vi "Measurement UI.vi"() -> ()   [LabVIEW 2021, in "Stepped Frequency Sweep_Class D Amplifier.lvlib"]
uses:
  Stepped Frequency Sweep_Class D Amplifier.lvlib
panel:
  in  "Graphs":T1(tab)
  out "Time domain graph":waveform(dbl)(graph)
  out "Sweep graph":T2(graph)
  out "Frequency domain graph":T3(graph)
  out "Output power (W)":dbl[](array[numeric])
  out "SFDR (dB)":dbl[](array[numeric])
  out "Gain error (dB)":dbl[](array[numeric])
  out "Dynamic range (dB)":dbl[](array[numeric])
  out "THD (dB)":dbl[](array[numeric])
  out "THD+N (dB)":dbl[](array[numeric])
  out "SNR (dB)":dbl[](array[numeric])
  out "Calculated amplitude (dB)":dbl[](array[numeric])
  out "Calculated frequency (Hz)":dbl[](array[numeric])
  in  "Configuration tab":enum32{"Protocol", "Measurement"}(tab)
  in  "master clock channel list":string caption="Master Clock Channel"
  in  "digital channel list":string caption="Digital Audio Channel"
  in  "logic level":enum32{"3.3 V", "1.8 V", "1.2 V"}(ring) caption="Logic level"
  in  "master clock rate":dbl=12288000.0 caption="Master clock rate" format="%#_6pHz"
  out "Bit clock rate":dbl=3072000.0 format="%#_6pHz"
  in  "number of channels":u8=2 caption="Number of channels"
  in  "TDM":bool
  in  "RJ":bool
  in  "LJ":bool
  in  "I2S":bool
  in  "bit clock edge sync":enum32{"Rising", "Falling"}(ring)=enum."Falling" caption="Bit clock edge sync"
  in  "frame clock rate":dbl=48000.0 caption="Frame clock rate" format="%#_6pHz"
  in  "data justification":enum32{"Left Justified", "Right Justified"}(ring) caption="Data justification"
  in  "endianness":enum32{"MSB First", "LSB First"}(ring) caption="Endianness"
  in  "bit depth":u8=24 caption="Bit depth"
  in  "channel length":u16=32 caption="Channel length"
  in  "frame sync edge for channel 0":enum32{"Rising", "Falling"}(ring)=enum."Falling" caption="Frame sync edge for Channel 0"
  in  "min settling cycles":u32 caption="Minimum settling cycles"
  in  "min settling time (s)":dbl=0.1 caption="Minimum settling time" format="%#_6ps"
  in  "sweep profile":enum16{"Linear", "Logarithmic"}(ring)=enum."Logarithmic" caption="Profile"
  in  "number of steps":u32=20000 caption="Number of steps"
  in  "sweep start frequency (Hz)":dbl=20.0 caption="Sweep start" format="%#_6pHz"
  in  "sweep stop frequency (Hz)":dbl=20000.0 caption="Sweep stop" format="%#_6pHz"
  in  "output power (W)":dbl=1.0 caption="Output power" format="%#_6p W"
  in  "output mode":enum16{"Level", "Power"}(ring) caption="Output mode"
  in  "min measurement cycles":u32 caption="Minimum measurement cycles"
  in  "Acquisition channel":tag
  in  "acq sampling rate":dbl=51200.0 caption="Sample rate" format="%#.6pHz"
  in  "min measurement time (s)":dbl=0.1 caption="Minimum measurement time" format="%#_6ps"
  in  "lowpass filter":T4(ring) caption="Lowpass filter"
  in  "highpass filter":enum32{"DC", "AC"}(ring) caption="Highpass filter"
  in  "band start":dbl=20.0 caption="Band start" format="%#_6pHz"
  in  "band stop":dbl=20000.0 caption="Band stop" format="%#_6pHz"
  in  "weighting filter":T5(ring)=enum."A-weighting" caption="Weighting filter"
  in  "load impedance":dbl=4.0 caption="Load impedance" format="%#_6p Ohms"
  in  "output range (pk-pk)":dbl=15.0 caption="Output range" format="%.3p Vpk-pk"
  in  "output level (dB)":dbl=-1.0 caption="Output level" format="%#_6p dBFS"
  in  "channel 0 offset":u32=1
  out "fft - data":dbl[](array[numeric])
  out "fft - df":dbl
  out "fft - f0":dbl
  out "wfm - data":dbl[](array[numeric])
  out "wfm - dt":dbl
  out "wfm - t0":dbl
  out "Channel name":string
  in  "acq channel":string="PXI1Slot4/ai0"
  in  "signal phase":dbl caption="phase"
  # "hidden controls - used to sync with MeasLink"
  # "hidden indicators"
  # "Protocols"
  # "Audio Protocol"
  # "Clock Settings"
  # "Signal Level"
  # "Harware Resource"
  # "Sweep"
  # "Filters"
  # "Output"
  # "Acquisition"
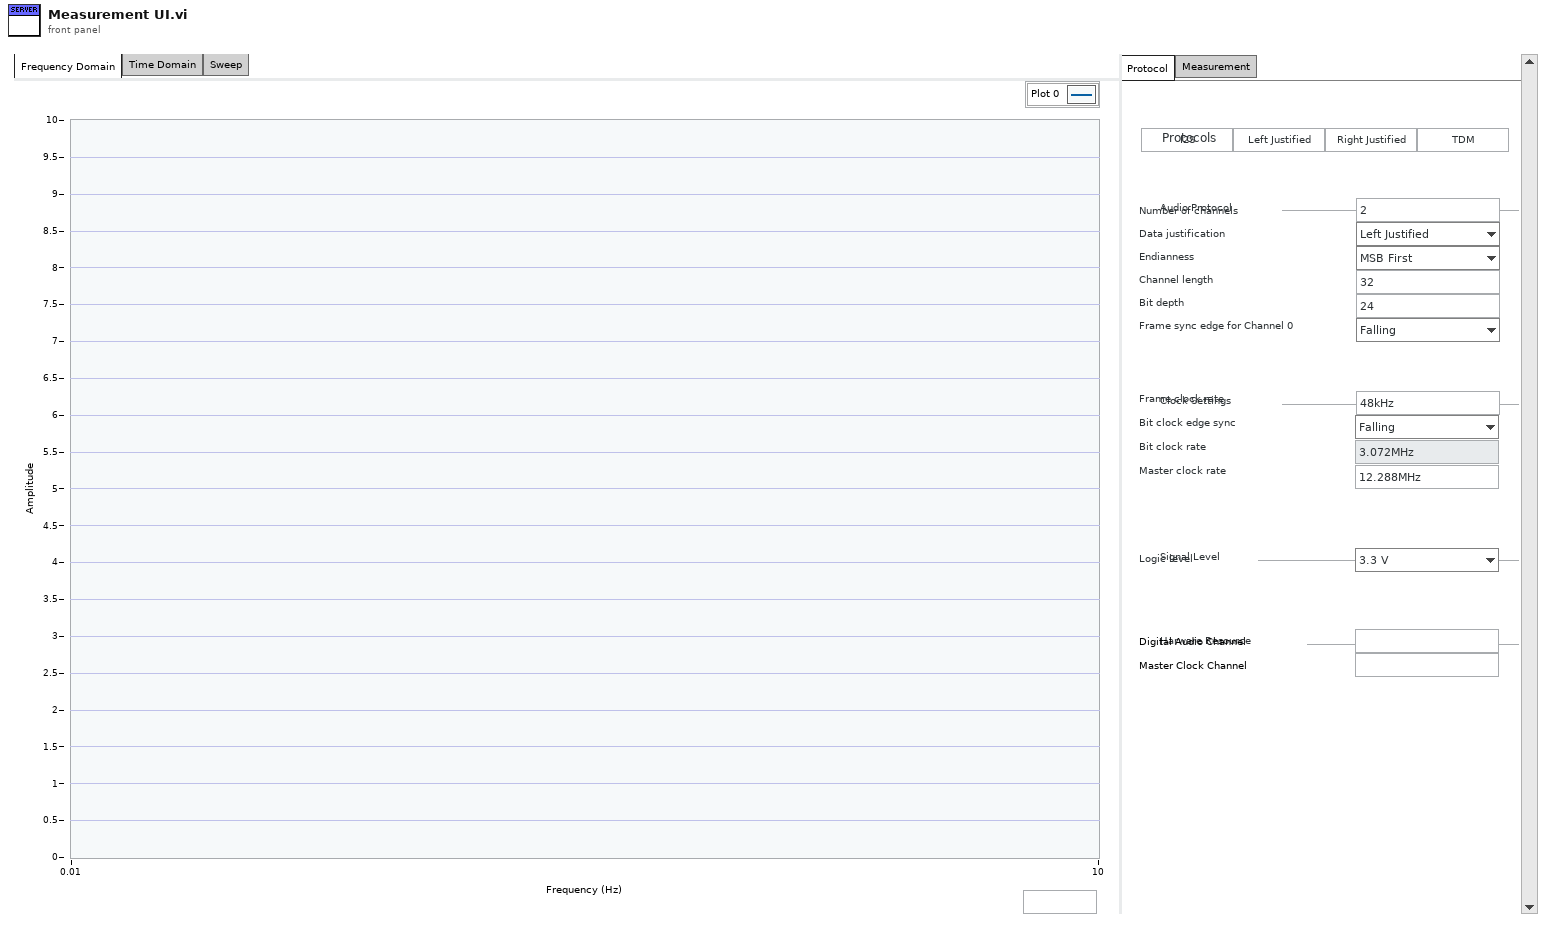
[diagram p1: front panel]
types:
  T1 = enum32{"Frequency Domain", "Time Domain", "Sweep"}
  T2 = cluster{"Calculated frequency (Hz)":dbl[], "THD+N (dB)":dbl[]}
  T3 = cluster{"fft - f0":dbl, "fft - df":dbl, "fft - data":dbl[]}
  T4 = enum32{"No filter", "AES17 20kHz", "AES17 40kHz"}
  T5 = enum32{"Linear", "A-weighting", "B-weighting", "C-weighting"}
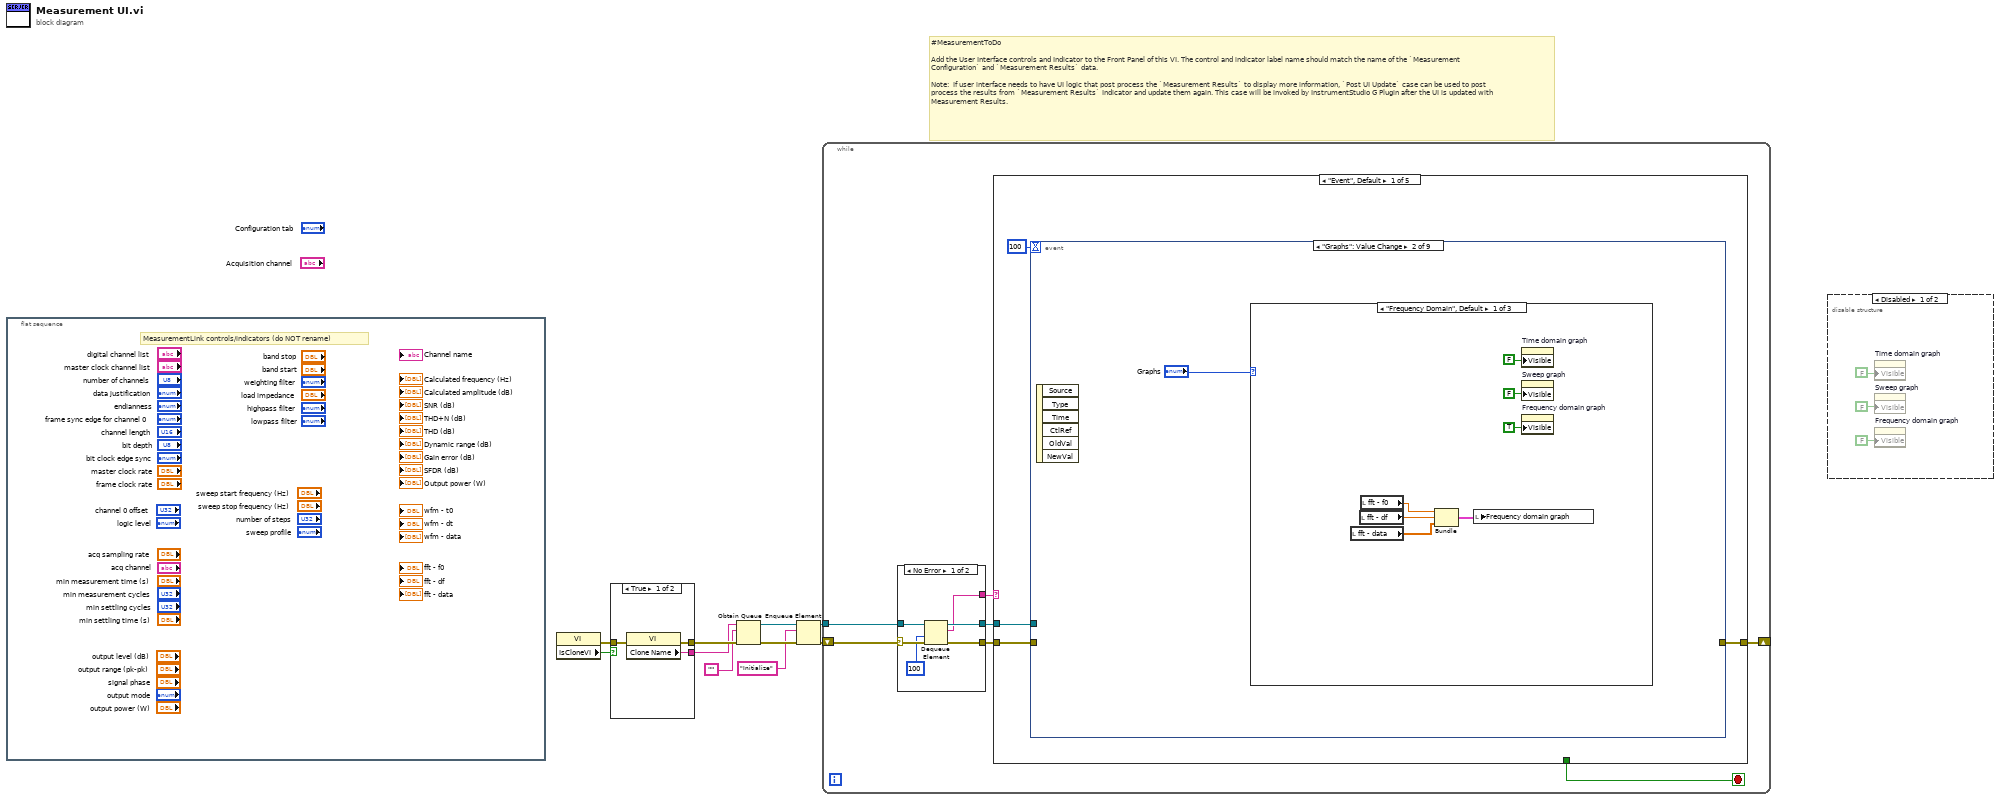
[diagram p0: block diagram]
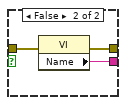
[diagram p3: hidden frame]
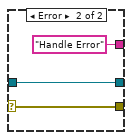
[diagram p4: hidden frame]
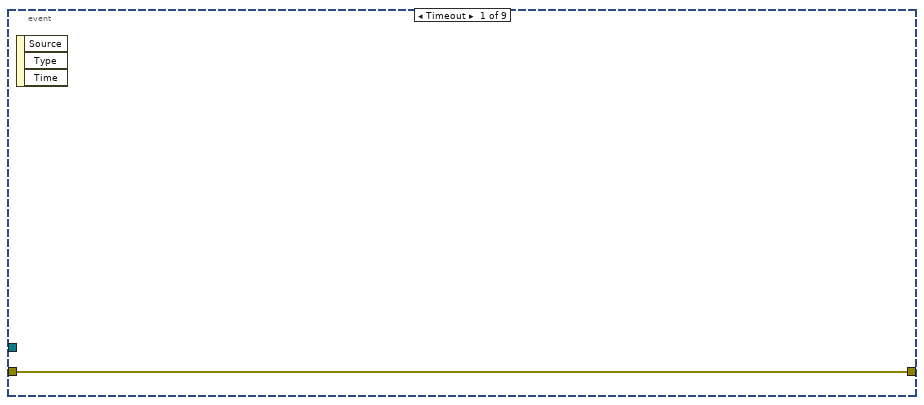
[diagram p5: hidden frame]
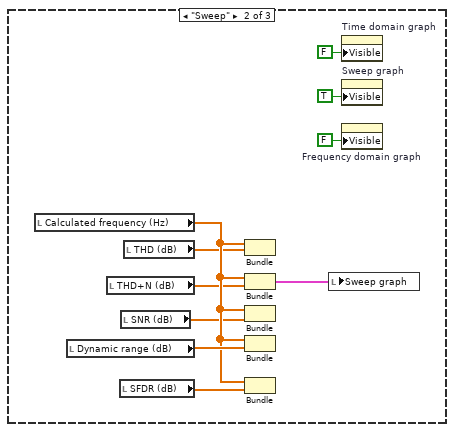
[diagram p6: hidden frame]
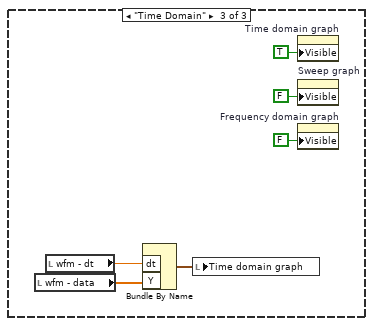
[diagram p7: hidden frame]
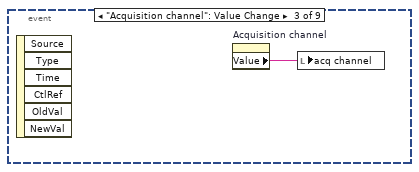
[diagram p8: hidden frame]
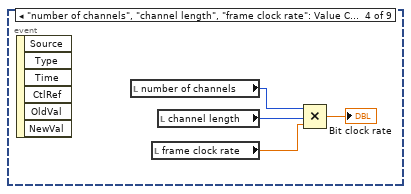
[diagram p9: hidden frame]
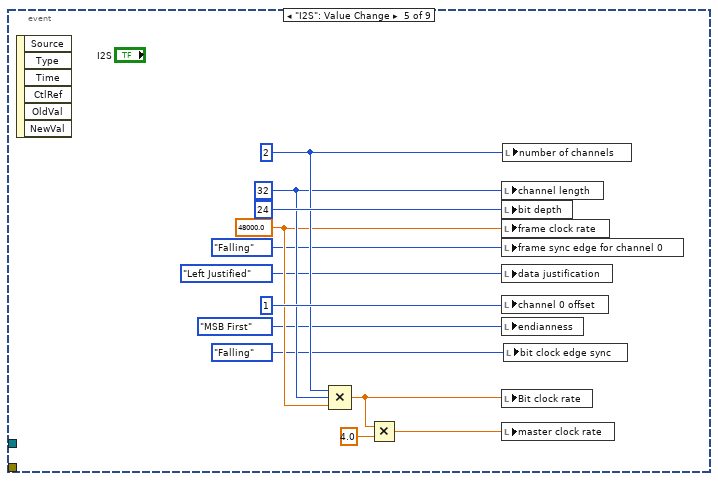
[diagram p10: hidden frame]
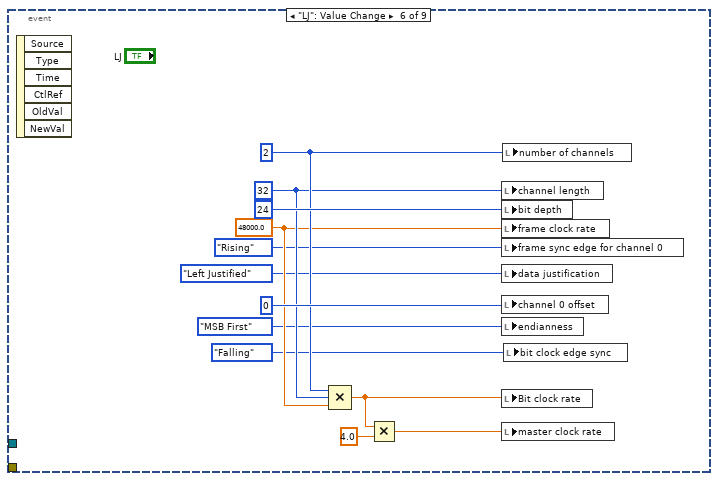
[diagram p11: hidden frame]
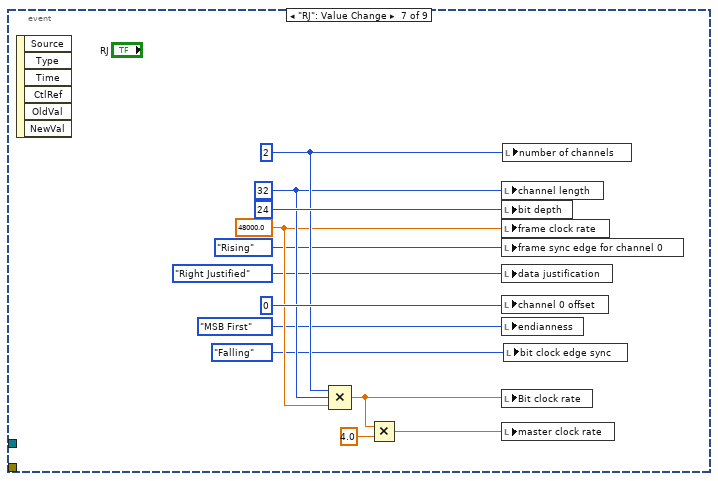
[diagram p12: hidden frame]
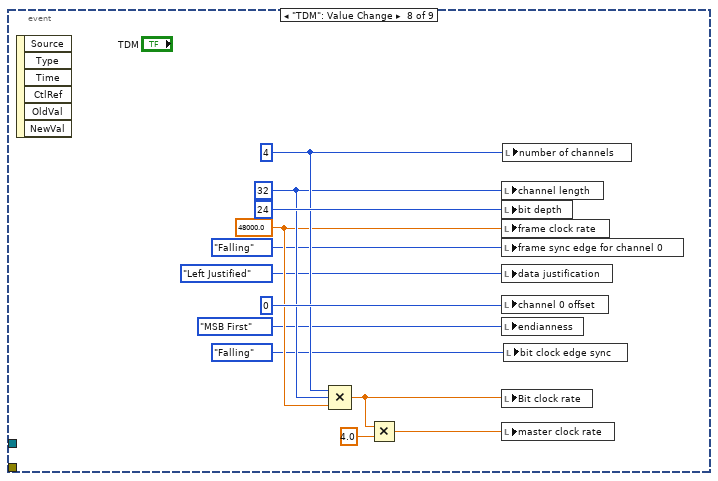
[diagram p13: hidden frame]
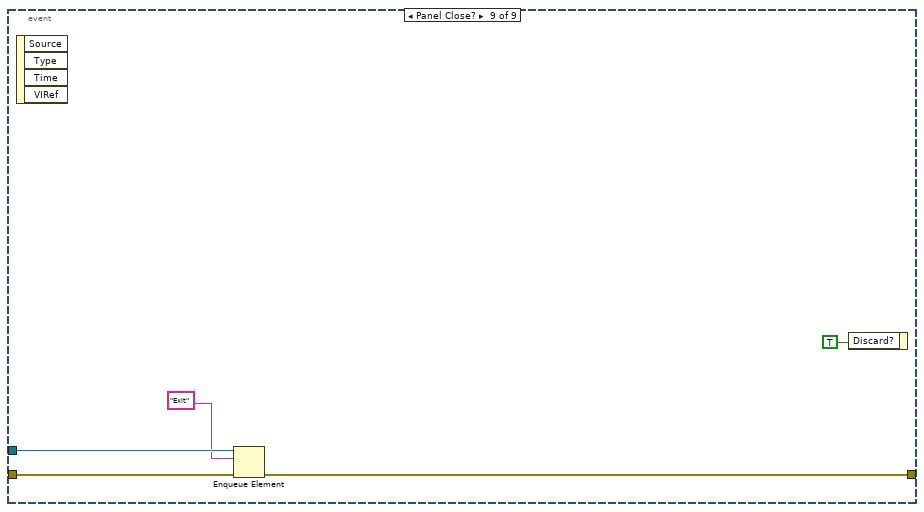
[diagram p14: hidden frame]
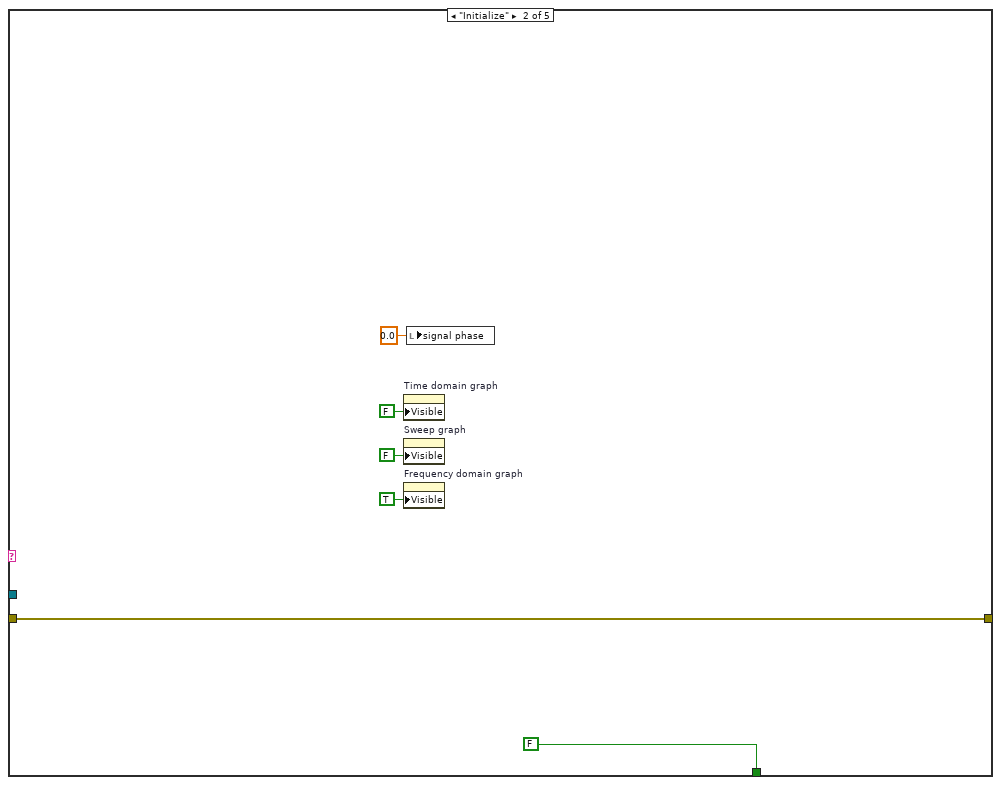
[diagram p15: hidden frame]
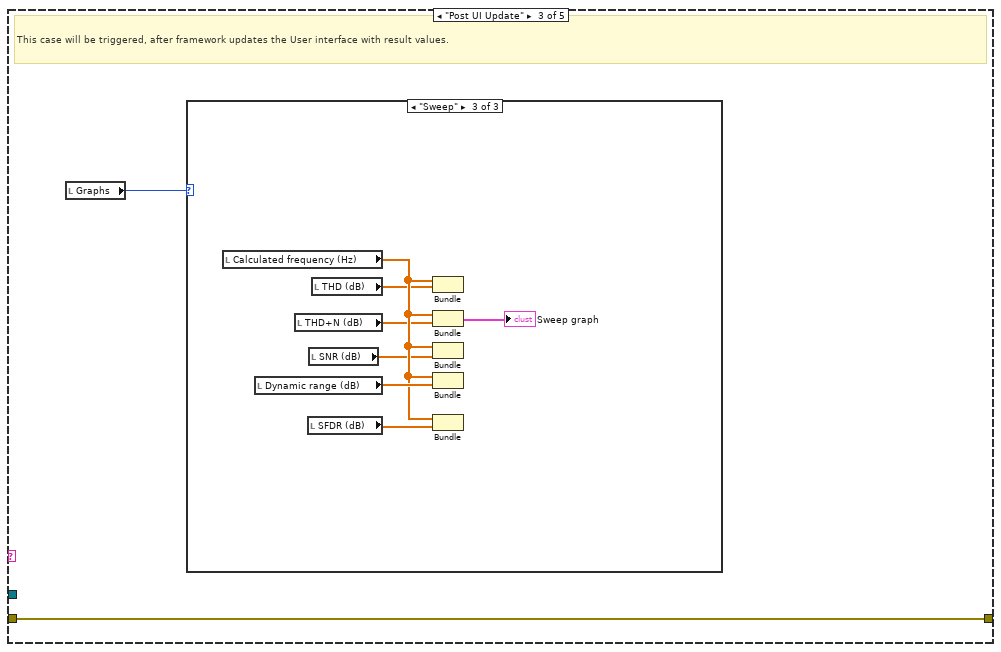
[diagram p16: hidden frame]
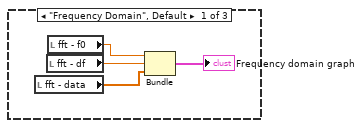
[diagram p17: hidden frame]
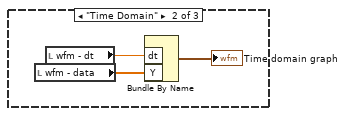
[diagram p18: hidden frame]
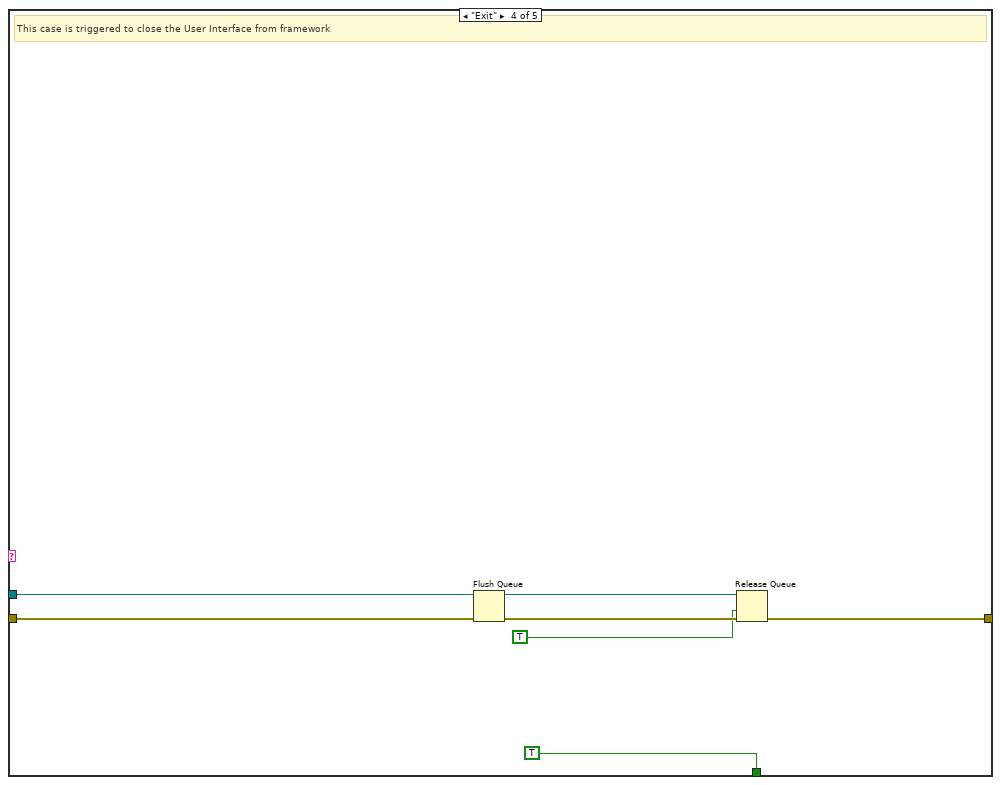
[diagram p19: hidden frame]
diagram:
  # "#MeasurementToDo  \n\nAdd the User Interface controls and Indicator to the Front Panel of this VI. The control and indicator label name should match the name of the `Measurement Configuration` and `Measurement Results` data.\n\nNote:  If user interface needs to have UI logic that post process the `Measurement Results` to display more information, `Post UI Update` case can be used to post process the results from `Measurement Results` Indicator and update them again. This case will be invoked by InstrumentStudio G Plugin after the UI is updated with Measurement Results."
  n1 = flat-sequence {
    frame #0 {
      # "MeasurementLink controls/indicators (do NOT rename)"
    }
  }
  n2 = property class="VI"() -> (error out=w1:errorcluster, "IsCloneVI"=w2:bool)  [unwired: 2 in, 1 out]
  n3 = case shown="True" w2 {
    tunnel: [w13 w16] -> w10
    tunnel: [w12 w15] -> w9
    tunnel: w1 -> [w11 w14]
    frame True {
      n4 = property class="VI"(error in=w11) -> (error out=w13:errorcluster, "Clone Name"=w12:string)  [unwired: 1 in, 1 out]
    }
    frame False {
      n5 = property class="VI"(error in=w14) -> (error out=w16:errorcluster, "Name"=w15:string)  [unwired: 1 in, 1 out]
    }
  }
  n6 = Obtain Queue(name (unnamed)=w9, element data type="", error in (no error)=w10) -> (queue out=w6:refnum<queue>, error out=w8:errorcluster)  [unwired: 2 in, 1 out]
  n7 = Enqueue Element(queue=w6, element="Initialize", error in (no error)=w8) -> (queue out=w5:refnum<queue>, error out=w7:errorcluster)  [unwired: 1 in, 1 out]
  n8 = while {
    shift-right: [w18] -> _
    shift-left: w7 -> [w23]
    tunnel: w5 -> [w21]
    stop <- w17 stop-if-true
    n9 = case shown="No Error" w23 {
      selector: w23 -> [w29 w32]
      tunnel: [w28 w32] -> w22
      tunnel: w21 -> [w27 w31]
      tunnel: [w26 w31] -> w20
      tunnel: [w25 "Handle Error"] -> w19
      frame No Error {
        n10 = Dequeue Element(queue=w27, timeout in ms (-1)=100, error in (no error)=w29) -> (queue out=w26:refnum<queue>, element=w25:string, error out=w28:errorcluster)  [unwired: 1 out]
      }
      frame Error {
      }
    }
    n11 = case shown="\"Event\", Default" w19 {
      tunnel: w22 -> [w35 w125 w127 w148 w149]
      tunnel: w20 -> [w33 _ _ w146 _]
      tunnel: [w36 w125 w127 w143 w149] -> w18
      tunnel: [_ FALSE _ TRUE _] -> w17
      frame "Event", Default {
        n12 = event shown="[1] \"Graphs\": Value Change" {
          selector: _ -> [_ _ _ _ _ _ _ _ _]
          dyn-events: _ -> [_ _ _ _ _ _ _ _ _]
          timeout: 100 -> [_ _ _ _ _ _ _ _ _]
          tunnel: [w37 _ _ _ _ _ _ _ w117] -> w36
          tunnel: w35 -> [w37 _ _ _ _ _ _ _ w118]
          tunnel: w33 -> [_ _ _ _ _ _ _ _ w116]
          event Timeout {
            n13 = event-data() -> ()  [unwired: 1 in, 3 out]
          }
          event "Graphs": Value Change {
            n14 = event-data() -> ()  [unwired: 1 in, 6 out]
            n15 = case shown="\"Frequency Domain\", Default" "Graphs" {
              frame "Frequency Domain", Default {
                n16 = local read "fft - data"() -> (w40:dbl[])
                n17 = local read "fft - df"() -> (w41:dbl)
                n18 = local read "fft - f0"() -> (w42:dbl)
                n19 = Bundle("fft - f0"=w42, "fft - df"=w41, "fft - data"=w40) -> (w39:T3)  [unwired: 1 in]
                n20 = local write "Frequency domain graph"(w39) -> ()
                n21 = property on="Time domain graph" class="WFGraph (strict)"("Visible"=FALSE) -> ()  [unwired: 2 in, 2 out]
                n22 = property on="Sweep graph" class="XYGraph (strict)"("Visible"=FALSE) -> ()  [unwired: 2 in, 2 out]
                n23 = property on="Frequency domain graph" class="WFGraph (strict)"("Visible"=TRUE) -> ()  [unwired: 2 in, 2 out]
              }
              frame "Sweep" {
                n24 = local read "Calculated frequency (Hz)"() -> (w50:dbl[])
                n25 = local read "Dynamic range (dB)"() -> (w52:dbl[])
                n26 = local read "THD+N (dB)"() -> (w48:dbl[])
                n27 = local read "SFDR (dB)"() -> (w51:dbl[])
                n28 = local read "SNR (dB)"() -> (w47:dbl[])
                n29 = local read "THD (dB)"() -> (w49:dbl[])
                n30 = Bundle("Calculated frequency (Hz)"=w50, "THD (dB)"=w49) -> ()  [unwired: 1 in, 1 out]
                n31 = Bundle("Calculated frequency (Hz)"=w50, "THD+N (dB)"=w48) -> (w46:T2)  [unwired: 1 in]
                n32 = Bundle("Calculated frequency (Hz)"=w50, "SNR (dB)"=w47) -> ()  [unwired: 1 in, 1 out]
                n33 = Bundle("Calculated frequency (Hz)"=w50, "Dynamic range (dB)"=w52) -> ()  [unwired: 1 in, 1 out]
                n34 = Bundle("Calculated frequency (Hz)"=w50, "SFDR (dB)"=w51) -> ()  [unwired: 1 in, 1 out]
                n35 = local write "Sweep graph"(w46) -> ()
                n36 = property on="Time domain graph" class="WFGraph (strict)"("Visible"=FALSE) -> ()  [unwired: 2 in, 2 out]
                n37 = property on="Sweep graph" class="XYGraph (strict)"("Visible"=TRUE) -> ()  [unwired: 2 in, 2 out]
                n38 = property on="Frequency domain graph" class="WFGraph (strict)"("Visible"=FALSE) -> ()  [unwired: 2 in, 2 out]
              }
              frame "Time Domain" {
                n39 = local read "wfm - data"() -> (w60:dbl[])
                n40 = local read "wfm - dt"() -> (w61:dbl)
                n41 = Bundle By Name("dt"=w61, "Y"=w60) -> (w59:waveform(dbl))  [unwired: 1 in]
                n42 = local write "Time domain graph"(w59) -> ()
                n43 = property on="Time domain graph" class="WFGraph (strict)"("Visible"=TRUE) -> ()  [unwired: 2 in, 2 out]
                n44 = property on="Sweep graph" class="XYGraph (strict)"("Visible"=FALSE) -> ()  [unwired: 2 in, 2 out]
                n45 = property on="Frequency domain graph" class="WFGraph (strict)"("Visible"=FALSE) -> ()  [unwired: 2 in, 2 out]
              }
            }
          }
          event "Acquisition channel": Value Change {
            n46 = event-data() -> ()  [unwired: 1 in, 6 out]
            n47 = property on="Acquisition channel" class="DAQmxName"() -> ("Value"=w62:string)  [unwired: 2 in, 2 out]
            n48 = local write "acq channel"(w62) -> ()
          }
          event "number of channels", "channel length", "frame clock rate": Value Change {
            n49 = event-data() -> ()  [unwired: 1 in, 6 out]
            n50 = local read "number of channels"() -> (w66:u8)
            n51 = local read "frame clock rate"() -> (w64:dbl)
            n52 = local read "channel length"() -> (w65:u16)
            n53 = Compound Arithmetic op=MULTIPLY(w66, w65, w64) -> (→"Bit clock rate":dbl)
          }
          event "I2S": Value Change {
            w74 = 48000.0 ("Frame Clock Rate")
            w75 = u32 32 ("Channel Length")
            w76 = u32 2 ("Number of Channels")
            n54 = event-data() -> ()  [unwired: 1 in, 6 out]
            n55 = Compound Arithmetic op=MULTIPLY(w76, w75, w74) -> (w73:dbl)
            n56 = Multiply(x=w73, y=4.0) -> (x*y=w72:dbl)
            n57 = local write "channel length"(w75) -> ()
            n58 = local write "bit depth"(u32 24 ("Bit Depth")) -> ()
            n59 = local write "frame clock rate"(w74) -> ()
            n60 = local write "frame sync edge for channel 0"(enum32{"Rising", "Falling"}."Falling" ("bit clock edge sync")) -> ()
            n61 = local write "data justification"(enum32{"Left Justified", "Right Justified"}."Left Justified" ("data justification")) -> ()
            n62 = local write "channel 0 offset"(u32 1 ("Channel 0 Offset")) -> ()
            n63 = local write "endianness"(enum32{"MSB First", "LSB First"}."MSB First" ("endianness")) -> ()
            n64 = local write "Bit clock rate"(w73) -> ()
            n65 = local write "master clock rate"(w72) -> ()
            n66 = local write "number of channels"(w76) -> ()
            n67 = local write "bit clock edge sync"(enum32{"Rising", "Falling"}."Falling" ("frame sync edge for channel 0")) -> ()
          }
          event "LJ": Value Change {
            w86 = 48000.0 ("Frame Clock Rate")
            w87 = u32 32 ("Channel Length")
            w88 = u32 2 ("Number of Channels")
            n68 = event-data() -> ()  [unwired: 1 in, 6 out]
            n69 = Compound Arithmetic op=MULTIPLY(w88, w87, w86) -> (w85:dbl)
            n70 = Multiply(x=w85, y=4.0) -> (x*y=w84:dbl)
            n71 = local write "channel length"(w87) -> ()
            n72 = local write "bit depth"(u32 24 ("Bit Depth")) -> ()
            n73 = local write "frame clock rate"(w86) -> ()
            n74 = local write "frame sync edge for channel 0"(enum32{"Rising", "Falling"}."Rising" ("bit clock edge sync")) -> ()
            n75 = local write "data justification"(enum32{"Left Justified", "Right Justified"}."Left Justified" ("data justification")) -> ()
            n76 = local write "channel 0 offset"(u32 0 ("Channel 0 Offset")) -> ()
            n77 = local write "endianness"(enum32{"MSB First", "LSB First"}."MSB First" ("endianness")) -> ()
            n78 = local write "Bit clock rate"(w85) -> ()
            n79 = local write "master clock rate"(w84) -> ()
            n80 = local write "number of channels"(w88) -> ()
            n81 = local write "bit clock edge sync"(enum32{"Rising", "Falling"}."Falling" ("frame sync edge for channel 0")) -> ()
          }
          event "RJ": Value Change {
            w98 = 48000.0 ("Frame Clock Rate")
            w99 = u32 32 ("Channel Length")
            w100 = u32 2 ("Number of Channels")
            n82 = event-data() -> ()  [unwired: 1 in, 6 out]
            n83 = Compound Arithmetic op=MULTIPLY(w100, w99, w98) -> (w97:dbl)
            n84 = Multiply(x=w97, y=4.0) -> (x*y=w96:dbl)
            n85 = local write "channel length"(w99) -> ()
            n86 = local write "bit depth"(u32 24 ("Bit Depth")) -> ()
            n87 = local write "frame clock rate"(w98) -> ()
            n88 = local write "frame sync edge for channel 0"(enum32{"Rising", "Falling"}."Rising" ("bit clock edge sync")) -> ()
            n89 = local write "data justification"(enum32{"Left Justified", "Right Justified"}."Right Justified" ("data justification")) -> ()
            n90 = local write "channel 0 offset"(u32 0 ("Channel 0 Offset")) -> ()
            n91 = local write "endianness"(enum32{"MSB First", "LSB First"}."MSB First" ("endianness")) -> ()
            n92 = local write "Bit clock rate"(w97) -> ()
            n93 = local write "master clock rate"(w96) -> ()
            n94 = local write "number of channels"(w100) -> ()
            n95 = local write "bit clock edge sync"(enum32{"Rising", "Falling"}."Falling" ("frame sync edge for channel 0")) -> ()
          }
          event "TDM": Value Change {
            w110 = 48000.0 ("Frame Clock Rate")
            w111 = u32 32 ("Channel Length")
            w112 = u32 4 ("Number of Channels")
            n96 = event-data() -> ()  [unwired: 1 in, 6 out]
            n97 = Compound Arithmetic op=MULTIPLY(w112, w111, w110) -> (w109:dbl)
            n98 = Multiply(x=w109, y=4.0) -> (x*y=w108:dbl)
            n99 = local write "channel length"(w111) -> ()
            n100 = local write "bit depth"(u32 24 ("Bit Depth")) -> ()
            n101 = local write "frame clock rate"(w110) -> ()
            n102 = local write "frame sync edge for channel 0"(enum32{"Rising", "Falling"}."Falling" ("bit clock edge sync")) -> ()
            n103 = local write "data justification"(enum32{"Left Justified", "Right Justified"}."Left Justified" ("data justification")) -> ()
            n104 = local write "channel 0 offset"(u32 0 ("Channel 0 Offset")) -> ()
            n105 = local write "endianness"(enum32{"MSB First", "LSB First"}."MSB First" ("endianness")) -> ()
            n106 = local write "Bit clock rate"(w109) -> ()
            n107 = local write "master clock rate"(w108) -> ()
            n108 = local write "number of channels"(w112) -> ()
            n109 = local write "bit clock edge sync"(enum32{"Rising", "Falling"}."Falling" ("frame sync edge for channel 0")) -> ()
          }
          event Panel Close? {
            n110 = event-data() -> ()  [unwired: 1 in, 4 out]
            n111 = Enqueue Element(queue=w116, element="Exit", error in (no error)=w118) -> (error out=w117:errorcluster)  [unwired: 1 in, 2 out]
            n112 = event-data("Discard?"=TRUE) -> ()  [unwired: 1 in, 1 out]
          }
        }
      }
      frame "Initialize" {
        n113 = property on="Time domain graph" class="WFGraph (strict)"("Visible"=FALSE) -> ()  [unwired: 2 in, 2 out]
        n114 = property on="Sweep graph" class="XYGraph (strict)"("Visible"=FALSE) -> ()  [unwired: 2 in, 2 out]
        n115 = property on="Frequency domain graph" class="WFGraph (strict)"("Visible"=TRUE) -> ()  [unwired: 2 in, 2 out]
        n116 = local write "signal phase"(0.0 ("signal phase")) -> ()
      }
      frame "Post UI Update" {
        # "This case will be triggered, after framework updates the User interface with result values."
        n117 = local read "Graphs"() -> (w126:T1)
        n118 = case shown="\"Sweep\"" w126 {
          frame "Frequency Domain", Default {
            n119 = local read "fft - data"() -> (w129:dbl[])
            n120 = local read "fft - df"() -> (w130:dbl)
            n121 = local read "fft - f0"() -> (w131:dbl)
            n122 = Bundle("fft - f0"=w131, "fft - df"=w130, "fft - data"=w129) -> (→"Frequency domain graph":T3)  [unwired: 1 in]
          }
          frame "Time Domain" {
            n123 = local read "wfm - data"() -> (w133:dbl[])
            n124 = local read "wfm - dt"() -> (w134:dbl)
            n125 = Bundle By Name("dt"=w134, "Y"=w133) -> (→"Time domain graph":waveform(dbl))  [unwired: 1 in]
          }
          frame "Sweep" {
            n126 = local read "Calculated frequency (Hz)"() -> (w139:dbl[])
            n127 = local read "Dynamic range (dB)"() -> (w141:dbl[])
            n128 = local read "THD+N (dB)"() -> (w137:dbl[])
            n129 = local read "SFDR (dB)"() -> (w140:dbl[])
            n130 = local read "SNR (dB)"() -> (w136:dbl[])
            n131 = local read "THD (dB)"() -> (w138:dbl[])
            n132 = Bundle("Calculated frequency (Hz)"=w139, "THD (dB)"=w138) -> ()  [unwired: 1 in, 1 out]
            n133 = Bundle("Calculated frequency (Hz)"=w139, "THD+N (dB)"=w137) -> (→"Sweep graph":T2)  [unwired: 1 in]
            n134 = Bundle("Calculated frequency (Hz)"=w139, "SNR (dB)"=w136) -> ()  [unwired: 1 in, 1 out]
            n135 = Bundle("Calculated frequency (Hz)"=w139, "Dynamic range (dB)"=w141) -> ()  [unwired: 1 in, 1 out]
            n136 = Bundle("Calculated frequency (Hz)"=w139, "SFDR (dB)"=w140) -> ()  [unwired: 1 in, 1 out]
          }
        }
      }
      frame "Exit" {
        # "This case is triggered to close the User Interface from framework"
        n137 = Flush Queue(queue=w146, error in (no error)=w148) -> (queue out=w145:refnum<queue>, error out=w144:errorcluster)  [unwired: 1 out]
        n138 = Release Queue(queue=w145, force destroy? (F)=TRUE, error in (no error)=w144) -> (error out=w143:errorcluster)  [unwired: 2 out]
      }
      frame "Handle Error" {
      }
    }
  }
  n139 = disable-structure shown="Disabled" {
    frame Disabled {
      n140 = property on="Time domain graph" class="WFGraph (strict)"("Visible"=FALSE) -> ()  [unwired: 2 in, 2 out]
      n141 = property on="Sweep graph" class="XYGraph (strict)"("Visible"=FALSE) -> ()  [unwired: 2 in, 2 out]
      n142 = property on="Frequency domain graph" class="WFGraph (strict)"("Visible"=FALSE) -> ()  [unwired: 2 in, 2 out]
    }
    frame Enabled {
    }
  }
